vi "Close XNET References.vi"(8 "error in (no error)":errorcluster, 11 "RT Configuration":T1 {"Frames"."Protection Configurations"."CRC Channels"."Data Type" items=["Signed", "Unsigned", "IEEE Float"]}) -> (0 "error out":errorcluster)   [LabVIEW 2015, in "Protection and Rolling Counter Addon Engine.lvlib"]
uses:
  Protection and Rolling Counter Addon Engine.lvlib
  Types/RT Async Engine Variables.ctl
  Types/RT Frame Settings.ctl
  Shared/Types/Exported Frame Type.ctl
  Types/RT Protection Configuration.ctl
  Shared/Types/Protection Type.ctl
  Shared/Types/InputChannelConfiguration.ctl
  Types/RT Counter Settings.ctl
  Shared/Types/Event Trigger Type.ctl
  Shared/Protection and Rolling Counter Addon Shared.lvlib
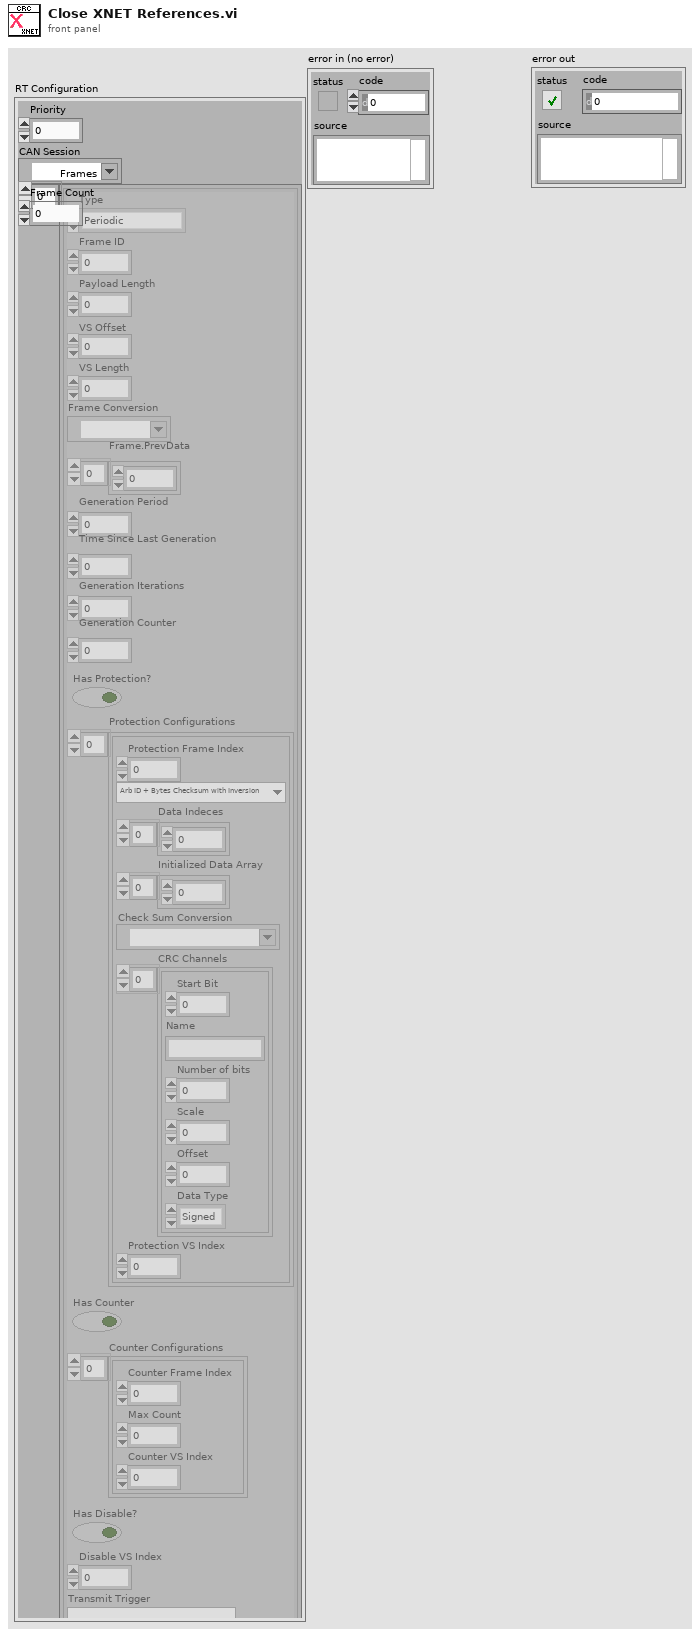
[diagram p1: front panel]
types:
  T1 = typedef "Protection and Rolling Counter Addon Engine.lvlib/RT Async Engine Variables.ctl" = cluster{"Priority":i32, "CAN Session":refnum<k21>, "Frame Count":i32, "Frames":T2[]}
  T2 = typedef "Protection and Rolling Counter Addon Engine.lvlib/RT Frame Settings.ctl" = cluster{"Type":T3, "Frame ID":u32, "Payload Length":u32, "VS Offset":i32, "VS Length":i32, "Frame Conversion":refnum<k21>, "Frame.PrevData":dbl[], "Generation Period":u32, "Time Since Last Generation":u32, "Generation Iterations":u32, "Generation Counter":u32, "Has Protection?":bool, "Protection Configurations":T4[], "Has Counter":bool, "Counter Configurations":T7[], "Has Disable?":bool, "Disable VS Index":i32, "Transmit Trigger":T8, "Trigger VS Index":i32}
  T3 = typedef "Exported Frame Type.ctl" = enum16{"Periodic", "Event"}
  T4 = typedef "Protection and Rolling Counter Addon Engine.lvlib/RT Protection Configuration.ctl" = cluster{"Protection Frame Index":i32, "Protection Type":T5, "Data Indeces":i32[], "Initialized Data Array":dbl[], "Check Sum Conversion":refnum<k21>, "CRC Channels":T6[], "Protection VS Index":i32}
  T5 = typedef "Protection and Rolling Counter Addon Shared.lvlib/Protection Type.ctl" = enum16{"Arb ID + Bytes Checksum with Inversion", "Arb ID + Bytes CRC with Inversion", "Reversed Raw Signal Checksum with Inversion"}
  T6 = typedef "Protection and Rolling Counter Addon Shared.lvlib/InputChannelConfiguration.ctl" = cluster{"Start Bit":i32, "Name":string, "Number of bits":i32, "Scale":dbl, "Offset":dbl, "Data Type":u32}
  T7 = typedef "Protection and Rolling Counter Addon Engine.lvlib/RT Counter Settings.ctl" = cluster{"Counter Frame Index":i32, "Max Count":dbl, "Counter VS Index":i32}
  T8 = typedef "Protection and Rolling Counter Addon Shared.lvlib/Event Trigger Type.ctl" = enum16{"Channel value change", "Trigger channel (not zero)", "Channel value change or trigger channel (not zero)", "Trigger channel (any value change)", "Channel value change or trigger channel (any value change)"}
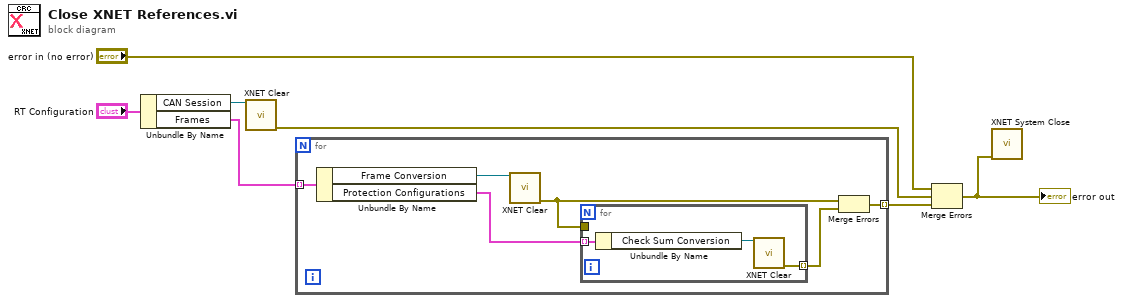
[diagram p0: block diagram]
diagram:
  n1 = Unbundle By Name("RT Configuration") -> ("CAN Session"=w6:refnum<k21>, "Frames"=w7:T2[])
  n2 = call <vilib>:"XNET Clear.vi"("session in"=w6) -> ("error out"=w3:errorcluster)  [unwired: 14 in]
  n3 = for {
    tunnel: w7 -> [w13] mode=indexing
    tunnel: [w8] -> w4 mode=indexing
    n4 = Unbundle By Name(w13) -> ("Frame Conversion"=w12:refnum<k21>, "Protection Configurations"=w11:T4[])
    n5 = call <vilib>:"XNET Clear.vi"("session in"=w12) -> ("error out"=w10:errorcluster)  [unwired: 14 in]
    n6 = for {
      tunnel: w11 -> [w16] mode=indexing
      tunnel: [w14] -> w9 mode=indexing
      tunnel: w10 -> [_]
      n7 = Unbundle By Name(w16) -> ("Check Sum Conversion"=w15:refnum<k21>)
      n8 = call <vilib>:"XNET Clear.vi"("session in"=w15) -> ("error out"=w14:errorcluster)  [unwired: 14 in]
    }
    n9 = Merge Errors(w10, w9) -> (w8:errorcluster)
  }
  n10 = Merge Errors("error in (no error)", w3, w4) -> (w1:errorcluster)
  "error out" <- w1
  n11 = call <vilib>:"XNET System Close.vi"("error in (no error)"=w1) -> ()  [unwired: 14 in, 1 out]
